vi "Simple-Calculator.vi"() -> ()   [LabVIEW 2014]
panel:
  in  "stop":bool
  out "Result":dbl
  in  "Enum":enum16{"Add", "Subtract", "Multiple", "Divide"}(ring)
  in  "Number 2":dbl
  in  "Number 1":dbl
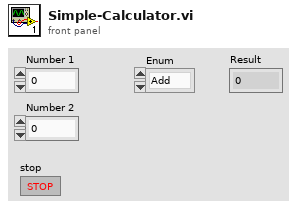
[diagram p1: front panel]
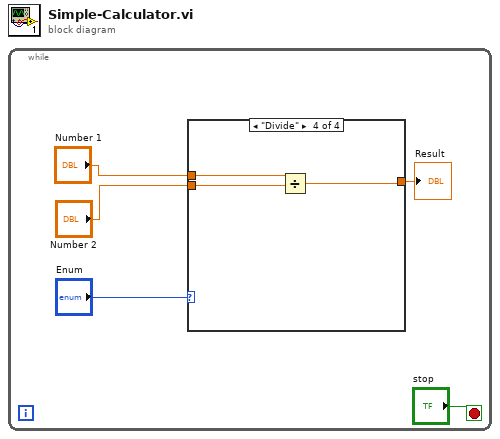
[diagram p0: block diagram]
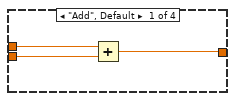
[diagram p2: hidden frame]
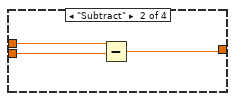
[diagram p3: hidden frame]
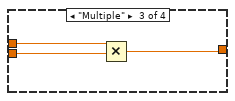
[diagram p4: hidden frame]
diagram:
  n1 = while {
    stop <- "stop" stop-if-true
    n2 = case shown="\"Divide\"" "Enum" {
      tunnel: "Number 1" -> [w8 w11 w14 w17]
      tunnel: "Number 2" -> [w7 w10 w13 w16]
      tunnel: [w6 w9 w12 w15] -> w2
      frame "Add", Default {
        n3 = Add(x=w8, y=w7) -> (x+y=w6:dbl)
      }
      frame "Subtract" {
        n4 = Subtract(x=w11, y=w10) -> (x-y=w9:dbl)
      }
      frame "Multiple" {
        n5 = Multiply(x=w14, y=w13) -> (x*y=w12:dbl)
      }
      frame "Divide" {
        n6 = Divide(x=w17, y=w16) -> (x/y=w15:dbl)
      }
    }
    "Result" <- w2
  }
